vi "USRP (transmitter,4800).vi"() -> ()   [LabVIEW 2013]
uses:
  IS-95/transmitter/4800/coding(4800).vi
  IS-95/transmitter/common/interleaver.vi
  IS-95/transmitter/9600/coding(9600).vi
  <vilib>/Analysis/baseanly.llb/A x B.vi
  <vilib>/Analysis/baseanly.llb/Real A x B.vi
  IS-95/transmitter/4800/syndrom(4800).vi
  IS-95/transmitter/9600/syndrom(9600).vi
  <instrlib>/niUSRP/niUSRP Write Tx Data (CDB).vi
  <vilib>/Analysis/Matrix/Numeric/Conversions/Array To Matrix.vi
  <vilib>/Analysis/Matrix/Numeric/Conversions/Array To Matrix - RA.vi
panel:
  in  "num of channels":i32=12
  in  "IQ rate":dbl=1000000.0 format="%#_13g"
  out "transmitted bits":bool[][](array[boolean])
  in  "device name":refnum<k15>="192.168.10.3"
  in  "gain":dbl=21.0 format="%#_6f"
  in  "carrier freq.":dbl=850000000.0 format="%#_6p"
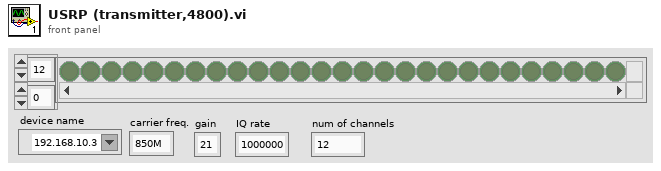
[diagram p1: front panel]
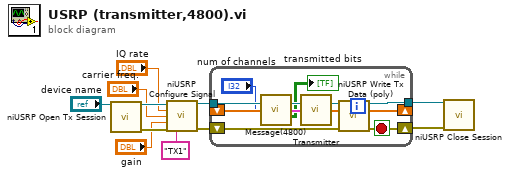
[diagram p0: block diagram]
diagram:
  n1 = call <instrlib>:"niUSRP Open Tx Session.vi"("device names"="device name") -> ("session handle out"=w11:refnum<k15>, "error out"=w10:errorcluster)  [unwired: 13 in]
  n2 = call <instrlib>:"niUSRP Configure Signal.vi"("session handle"=w11, "IQ rate"="IQ rate", "carrier frequency"="carrier freq.", "gain"="gain", "error in (no error)"=w10, "active antenna"="TX1") -> ("session handle out"=w4:refnum<k15>, "error out"=w3:errorcluster)  [unwired: 5 in, 3 out]
  n3 = while {
    tunnel: w4 -> [w20]
    shift-right: [w17] -> w1
    shift-left: w3 -> [w18]
    tunnel: [w19] -> w2
    shift-right: [w15] -> _
    shift-left: _ -> [w14]
    stop <- w17 stop-if-true
    n4 = call "Message(4800).vi"("num of channels"="num of channels") -> ("Channels"=w16:cluster{dbl, i32, bool[], "Type":i32}[], "Message"=→"transmitted bits":bool[][])  [unwired: 13 in]
    n5 = call "Transmitter.vi"("CHANNELS"=w16) -> ("x + iy"=w15:cdb[])  [unwired: 14 in]
    n6 = call-poly <instrlib>:"niUSRP Write Tx Data (poly).vi"("session handle"=w20, "data"=w14, "error in (no error)"=w18) -> ("session handle out"=w19:refnum<k15>, "error out"=w17:errorcluster)  [unwired: 11 in]
  }
  n7 = call <instrlib>:"niUSRP Close Session.vi"("session handle"=w2, "error in (no error)"=w1) -> ()  [unwired: 13 in, 1 out]
